vi "KlingerV2 Goto.vi"(0 "VISA Rsrc":refnum<visa-resource-name>="SR530", 1 "Ctrl Refs":T1, 5 "Relatif":bool caption="Relatif/Absolu\n(Absolu)", 7 "UnitDem":u8(ring)=2 caption="Unités" items=["Pas", "mm", "ps"], 9 "PosDem":dbl=1.0 caption="Position dem (pas)" min=-7999999.9 max=7999999.9 step=0.1 format="%#_8f", 11 "error in":errorcluster, 12 "Axe":u8(ring) items=["W", "X", "Y", "Z"]) -> (3 "Erreur":bool, 4 "Pos Init":dbl caption="Position Initiale", 6 "PosErreur":dbl caption="Erreur de\nPositionnement", 8 "Limits":cluster{"PLimit":bool, "NLimit":bool}, 10 "Position Out":dbl format="%#.3f", 14 "Indcomm":string caption="Indicateur de commande", 15 "error out":errorcluster)   [LabVIEW 2019]
doc: "Ce VI envoie une commande de déplacement au controlleur Klinger MC4. \n\nAxe : Sélectionner l'axe sur lequel effectuer le déplacement\n\nAllez à :En mode de déplacement absolu, entrer la position de destination en pas. En mode de déplacement relatif, entrer le nombre de pas à effectuer. Le signe indique la direcetion de déplacement. Valeur accepter :-7 999 999,9 à 7 999 999,9\n\nRelatif/Absolu : Choisi le type de déplacementà effectuer. En mode absolu, le déplacement est effectué par rapport à une position de référence prédéfini. En mode relatif, le déplacement est effectué par rapport à la position actuelle.\n\nLimite + : Indique l'atteinte de l'interrupeur de fin de course positif\n\nLimite - : Indique l'atteinte de l'interrupeur de fin de course négatif\n\nPosition: Indique la position finale"
uses:
  <userlib>/KlingerV2/KlingerV2 Params.ctl
  <userlib>/KlingerV2/KlingerV2 GotoStates.ctl
  <vilib>/Utility/error.llb/DialogType.ctl
panel:
  out "Stopped":bool
  out "NbEssais":i32
  out "Message D'erreur":string
  out "Moving":bool caption="Déplacement\nen cours"
  # "Relatif"
  # "Absolu"
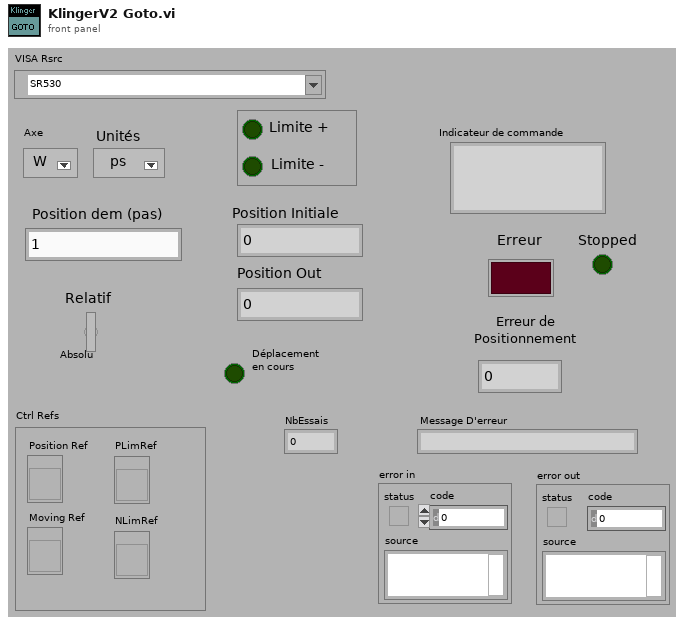
[diagram p1: front panel]
types:
  T1 = cluster{"Position Ref":refnum<vi>, "Moving Ref":refnum<vi>, "PLimRef":refnum<vi>, "NLimRef":refnum<vi>}
  T2 = typedef "KlingerV2 GotoStates.ctl" = enum16{"Dem Pos Init", "Lire Pos Init", "Envoie Comm", "Dem Statut", "Lire Statut", "Attend RQS", "Erreur GPIB", "Dépl incomp", "StopMove", "Dépl comp"}
  T3 = typedef "KlingerV2 Params.ctl" = enum16{"Type", "Origine", "Encodeur", "TypeMouv", "FactConv", "Nom", "CorrParams", "KlingCtrlPar", "Speed", "Acc", "Avance", "Tous"}
  T4 = cluster{"CorrActive":bool, "ErreurLim":dbl, "NbrEssais":i32}
  T5 = typedef "DialogType.ctl" = u16
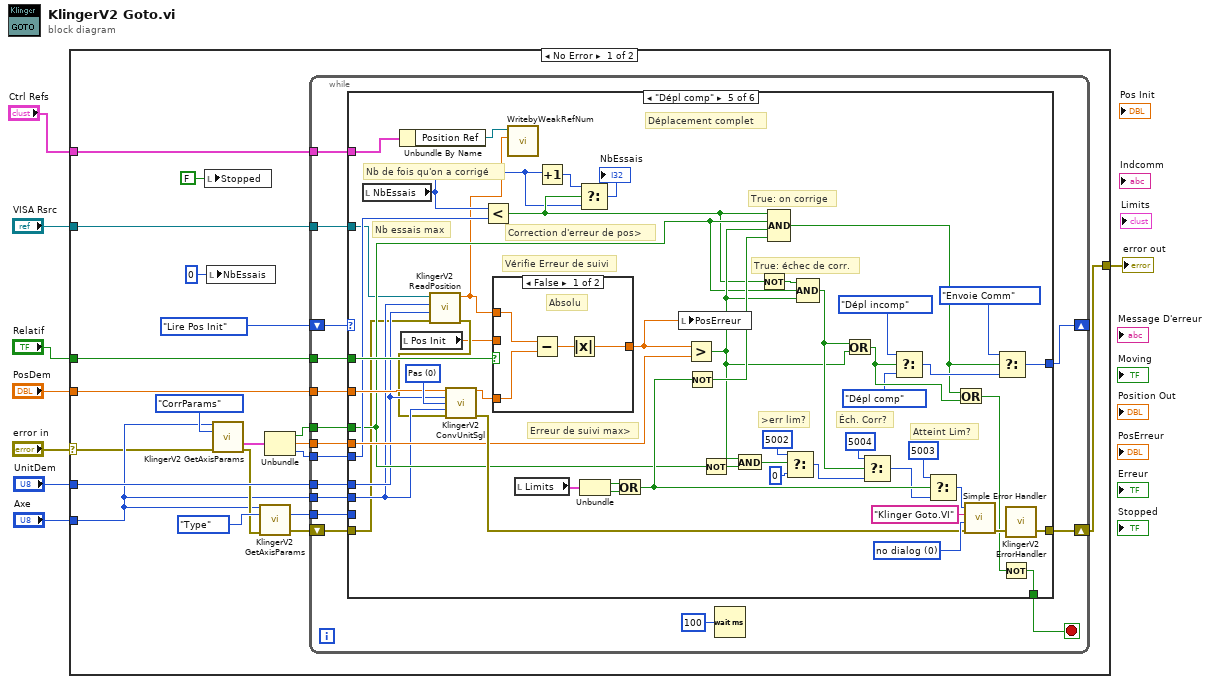
[diagram p0: block diagram]
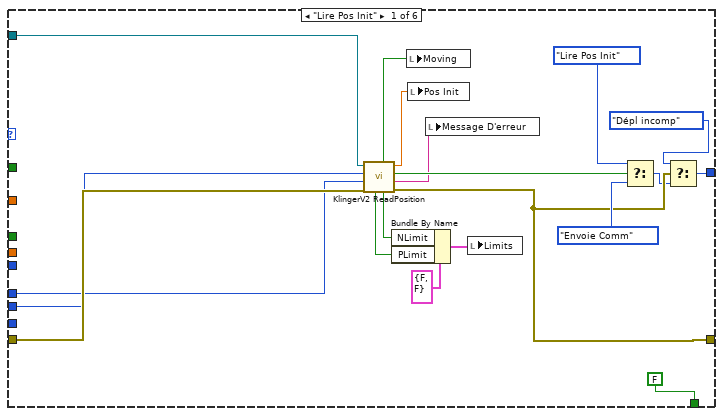
[diagram p2: hidden frame]
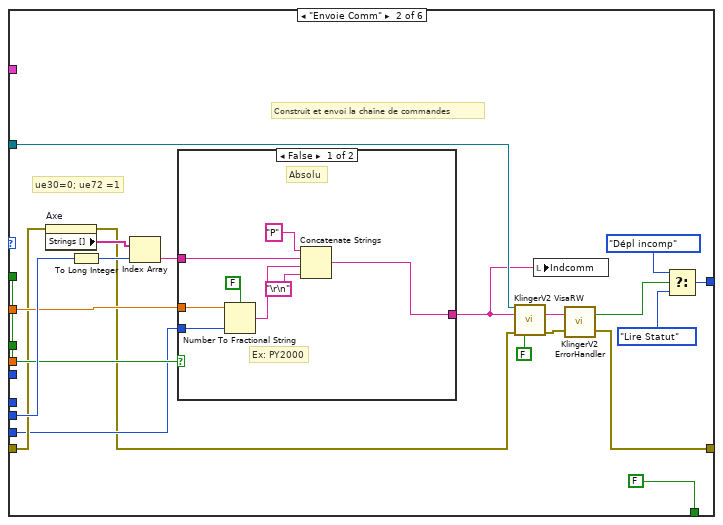
[diagram p3: hidden frame]
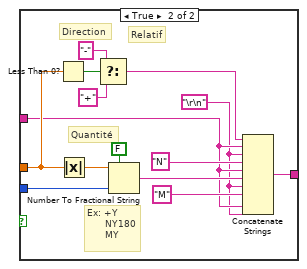
[diagram p4: hidden frame]
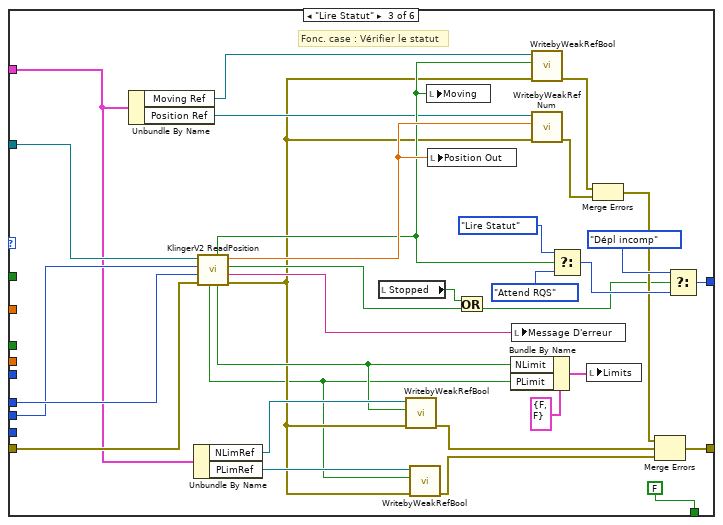
[diagram p5: hidden frame]
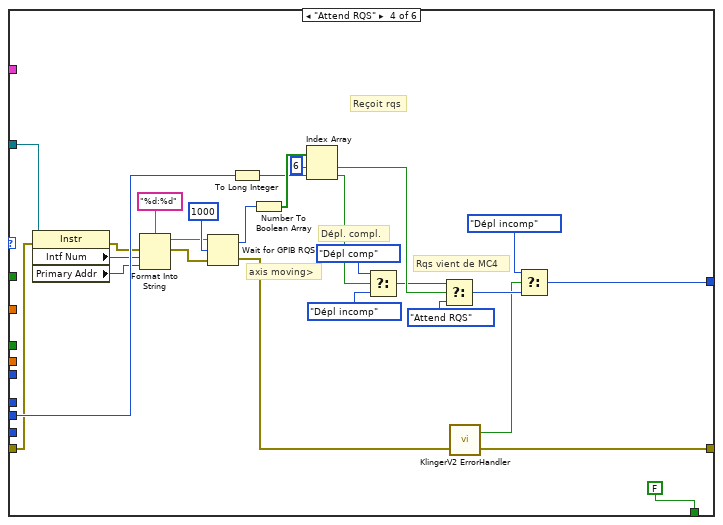
[diagram p6: hidden frame]
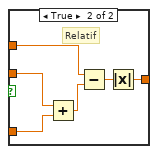
[diagram p7: hidden frame]
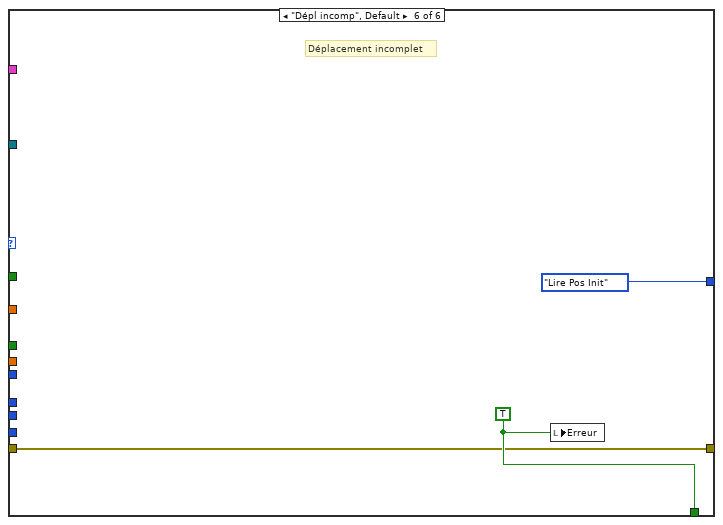
[diagram p8: hidden frame]
diagram:
  n1 = case shown="No Error" "error in" {
    selector: "error in" -> [w10 w230]
    tunnel: [w28 w230] -> w8
    tunnel: "UnitDem" -> [w21 _]
    tunnel: "PosDem" -> [w20 _]
    tunnel: "Relatif" -> [w19 _]
    tunnel: "Axe" -> [w11 _]
    tunnel: "VISA Rsrc" -> [w9 _]
    tunnel: "Ctrl Refs" -> [w14 _]
    frame No Error {
      n2 = local write "Stopped"(FALSE ("Stopped")) -> ()
      n3 = local write "NbEssais"(0 ("Numeric")) -> ()
      n4 = call <userlib>:"KlingerV2 GetAxisParams.vi"("Axe"=w11, "Param"=KlingerV2_Params."CorrParams", "error in"=w10) -> ("CorrParams"=w18:T4, "error out"=w17:errorcluster)  [unwired: 3 in, 8 out]
      n5 = call <userlib>:"KlingerV2 GetAxisParams.vi"("Axe"=w11, "Param"=KlingerV2_Params."Type", "error in"=w17) -> ("Type"=w22:i32, "error out"=w16:errorcluster)  [unwired: 3 in, 8 out]
      n6 = Unbundle(w18) -> ("CorrActive"=w25:bool, "ErreurLim"=w26:dbl, "NbrEssais"=w24:i32)
      n7 = while {
        shift-right: [w43] -> w28
        shift-left: w16 -> [w42]
        tunnel: w11 -> [w41]
        tunnel: w20 -> [w40]
        tunnel: w19 -> [w39]
        shift-right: [w36] -> _
        shift-left: KlingerV2_GotoStates."Lire Pos Init" ("KlingerV2 GotoStates") -> [w37]
        tunnel: w24 -> [w35]
        tunnel: w21 -> [w34]
        tunnel: w26 -> [w33]
        tunnel: w25 -> [w32]
        tunnel: w22 -> [w31]
        tunnel: w9 -> [w30]
        tunnel: w14 -> [w29]
        stop <- w44 stop-if-true
        n8 = case shown="\"Dépl comp\"" w37 {
          tunnel: [FALSE FALSE FALSE FALSE w212 w229] -> w44
          tunnel: [w47 w76 w112 w138 w211 w228] -> w43
          tunnel: w42 -> [w60 w73 w133 w146 w168 w228]
          tunnel: w41 -> [w56 w80 w130 w164 w169 _]
          tunnel: w40 -> [_ w74 _ _ w203 _]
          tunnel: w39 -> [_ w78 _ _ w216 _]
          tunnel: [w48 w77 w136 w139 w204 KlingerV2_GotoStates."Lire Pos Init" ("KlingerV2 GotoStates")] -> w36
          tunnel: w35 -> [_ _ _ _ w179 _]
          tunnel: w34 -> [w57 _ w131 _ w170 _]
          tunnel: w33 -> [_ _ _ _ w189 _]
          tunnel: w32 -> [_ _ _ _ w178 _]
          tunnel: w31 -> [_ w72 _ _ _ _]
          tunnel: w30 -> [w58 w71 w127 w148 w173 _]
          tunnel: w29 -> [_ _ w120 _ w172 _]
          frame "Lire Pos Init" {
            n9 = call <userlib>:"KlingerV2 ReadPosition.vi"("error in"=w60, "UnitDem"=w57, "Axe"=w56, "VISA Rsrc"=w58) -> ("error out"=w47:errorcluster, "Cont Error"=w61:string, "Statut"=w62:bool, "Position"=w59:dbl, "NLimit"=w52:bool, "Moving"=w55:bool, "PLimit"=w53:bool)  [unwired: 1 in]
            n10 = Bundle By Name(cluster=cluster{"PLimit":bool, "NLimit":bool} {"PLimit"=FALSE, "NLimit"=FALSE} ("Limits"), "NLimit"=w52, "PLimit"=w53) -> (w51:cluster{"PLimit":bool, "NLimit":bool})
            n11 = local write "Moving"(w55) -> ()
            n12 = local write "Pos Init"(w59) -> ()
            n13 = local write "Message D'erreur"(w61) -> ()
            n14 = local write "Limits"(w51) -> ()
            n15 = Select(t=KlingerV2_GotoStates."Lire Pos Init" ("KlingerV2 GotoStates"), s=w62, f=KlingerV2_GotoStates."Envoie Comm" ("KlingerV2 GotoStates")) -> (s? t:f=w46:T2)
            n16 = Select(t=KlingerV2_GotoStates."Dépl incomp" ("KlingerV2 GotoStates"), s=w47, f=w46) -> (s? t:f=w48:T2)
          }
          frame "Envoie Comm" {
            # "ue30=0; ue72 =1"
            # "Construit et envoi la chaîne de commandes"
            n17 = property on="Axe" class="Ring (strict)"(error in=w73) -> (error out=w70:errorcluster, "Strings []"=w83:string[])  [unwired: 1 in, 1 out]
            n18 = To Long Integer(number=w80) -> (32bit integer=w79:i32)
            n19 = Index Array(array=w83, index=w79) -> (element=w82:string)
            n20 = case shown="False" w78 {
              tunnel: w74 -> [w91 w103]
              tunnel: w82 -> [w88 w95]
              tunnel: [w86 w93] -> w69
              tunnel: w72 -> [w84 w92]
              frame False {
                # "Ex: PY2000"
                # "Absolu"
                n21 = Number To Fractional String(use system decimal point (T)=FALSE, number=w91, precision (6)=w84) -> (F-format string=w90:string)  [unwired: 1 in]
                n22 = Concatenate Strings("P", w88, w90, "\r\n") -> (w86:string)
              }
              frame True {
                w94 = "\r\n"
                # "Quantité"
                # "Direction"
                # "Ex: +Y\n      NY180\n      MY"
                # "Relatif"
                n23 = Less Than 0?(x=w103) -> (x < 0?=w102:bool)
                n24 = Absolute Value(x=w103) -> (abs(x)=w105:dbl)
                n25 = Select(t="-", s=w102, f="+") -> (s? t:f=w99:string)
                n26 = Number To Fractional String(use system decimal point (T)=FALSE, number=w105, precision (6)=w92) -> (F-format string=w97:string)  [unwired: 1 in]
                n27 = Concatenate Strings(w99, w95, w94, "N", w95, w97, w94, "M", w95, w94) -> (w93:string)
              }
            }
            n28 = call <userlib>:"KlingerV2 VisaRW.vi"("VISA Rsrc"=w71, "ChaineCom"=w69, "error in (no error)"=w70, "Lecture?(T)"=FALSE) -> ("ChaineRep"=w67:string, "error out"=w68:errorcluster)  [unwired: 7 in, 3 out]
            n29 = local write "Indcomm"(w69) -> ()
            n30 = call <userlib>:"KlingerV2 ErrorHandler.vi"("error in (no error)"=w68, "Message D'erreur"=w67) -> ("error out"=w76:errorcluster, "Erreur"=w75:bool)
            n31 = Select(t=KlingerV2_GotoStates."Dépl incomp" ("KlingerV2 GotoStates"), s=w75, f=KlingerV2_GotoStates."Lire Statut" ("KlingerV2 GotoStates")) -> (s? t:f=w77:T2)
          }
          frame "Lire Statut" {
            # "Fonc. case : Vérifier le statut"
            n32 = Unbundle By Name(w120) -> ("Moving Ref"=w124:refnum<vi>, "Position Ref"=w123:refnum<vi>)
            n33 = Unbundle By Name(w120) -> ("NLimRef"=w119:refnum<vi>, "PLimRef"=w118:refnum<vi>)
            n34 = call <userlib>:"KlingerV2 ReadPosition.vi"("error in"=w133, "UnitDem"=w131, "Axe"=w130, "VISA Rsrc"=w127) -> ("error out"=w116:errorcluster, "Cont Error"=w132:string, "Statut"=w134:bool, "Position"=w129:dbl, "NLimit"=w117:bool, "Moving"=w128:bool, "PLimit"=w115:bool)  [unwired: 1 in]
            n35 = local read "Stopped"() -> (w107:bool)
            n36 = call <userlib>:"WritebyWeakRefBool.vi"("error in"=w116, "Valeur"=w117, "Control Ref"=w119) -> ("error out"=w110:errorcluster)  [unwired: 8 in]
            n37 = call <userlib>:"WritebyWeakRefBool.vi"("error in"=w116, "Valeur"=w115, "Control Ref"=w118) -> ("error out"=w109:errorcluster)  [unwired: 8 in]
            n38 = local write "Moving"(w128) -> ()
            n39 = local write "Position Out"(w129) -> ()
            n40 = Or(x=w107, y=w134) -> (x .or. y?=w108:bool)
            n41 = Bundle By Name(cluster=cluster{"PLimit":bool, "NLimit":bool} {"PLimit"=FALSE, "NLimit"=FALSE} ("Limits"), "NLimit"=w117, "PLimit"=w115) -> (w125:cluster{"PLimit":bool, "NLimit":bool})
            n42 = local write "Message D'erreur"(w132) -> ()
            n43 = call <userlib>:"WritebyWeakRefBool.vi"("error in"=w116, "Valeur"=w128, "Control Ref"=w124) -> ("error out"=w113:errorcluster)  [unwired: 8 in]
            n44 = call <userlib>:"WritebyWeakRefNum.vi"("error in"=w116, "Valeur"=w129, "Control Ref"=w123) -> ("error out"=w114:errorcluster)  [unwired: 8 in]
            n45 = Select(t=KlingerV2_GotoStates."Lire Statut" ("KlingerV2 GotoStates"), s=w128, f=KlingerV2_GotoStates."Attend RQS" ("KlingerV2 GotoStates")) -> (s? t:f=w135:T2)
            n46 = local write "Limits"(w125) -> ()
            n47 = Merge Errors(w113, w114) -> (w111:errorcluster)
            n48 = Merge Errors(w111, w110, w109) -> (w112:errorcluster)
            n49 = Select(t=KlingerV2_GotoStates."Dépl incomp" ("KlingerV2 GotoStates"), s=w108, f=w135) -> (s? t:f=w136:T2)
          }
          frame "Attend RQS" {
            # "axis moving>"
            # "Dépl. compl."
            # "Rqs vient de MC4"
            # "Reçoit rqs"
            n50 = property class="Instr"(reference=w148, error in=w146) -> (error out=w143:errorcluster, "Intf Num"=w145:u16, "Primary Addr"=w144:u16)  [unwired: 1 out]
            n51 = Format Into String(format string="%d:%d" ("chaîne de format"), error in=w143, w145, w144) -> (resulting string=w142:string, error out=w141:errorcluster)  [unwired: 1 in]
            n52 = Wait for GPIB RQS(2:w141, 3:1000 ("timeout (25000 ms)"), 4:w142) -> (0:w150:errorcluster, 1:w149:i16)
            n53 = To Long Integer(number=w164) -> (32bit integer=w159:i32)
            n54 = Number To Boolean Array(number=w149) -> (Boolean array=w163:bool[])
            n55 = Index Array(array=w163, index #1=6 ("index"), index #2=w159) -> (element #1=w161:bool, element #2=w158:bool)
            n56 = Select(t=KlingerV2_GotoStates."Dépl comp" ("KlingerV2 GotoStates"), s=w158, f=KlingerV2_GotoStates."Dépl incomp" ("KlingerV2 GotoStates")) -> (s? t:f=w157:T2)
            n57 = Select(t=w157, s=w161, f=KlingerV2_GotoStates."Attend RQS" ("KlingerV2 GotoStates")) -> (s? t:f=w156:T2)
            n58 = call <userlib>:"KlingerV2 ErrorHandler.vi"("error in (no error)"=w150) -> ("error out"=w138:errorcluster, "Erreur"=w155:bool)  [unwired: 1 in]
            n59 = Select(t=KlingerV2_GotoStates."Dépl incomp" ("KlingerV2 GotoStates"), s=w155, f=w156) -> (s? t:f=w139:T2)
          }
          frame "Dépl comp" {
            w210 = u8 0 items=["Pas", "mm", "ps"] ("UnitAct")
            w214 = T5 0 items=["no dialog", "OK message", "continue or stop message", "OK message + warnings", "continue/stop + warnings"] ("type of dialog (OK msg:1)")
            # "Nb essais max"
            # "Correction d'erreur de pos>"
            # "Erreur de suivi max>"
            # ">err lim?"
            # "Éch. Corr?"
            # "Atteint Lim?"
            # "Nb de fois qu'on a corrigé"
            # "True: échec de corr."
            # "True: on corrige"
            # "Vérifie Erreur de suivi"
            # "Déplacement complet"
            n60 = local read "NbEssais"() -> (w176:i32)
            n61 = Unbundle By Name(w172) -> ("Position Ref"=w171:refnum<vi>)
            n62 = local read "Pos Init"() -> (w166:dbl)
            n63 = call <userlib>:"KlingerV2 ReadPosition.vi"("error in"=w168, "UnitDem"=w170, "Axe"=w169, "VISA Rsrc"=w173) -> ("error out"=w167:errorcluster, "Position"=w165:dbl)  [unwired: 1 in, 5 out]
            n64 = call <userlib>:"KlingerV2 ConvUnitSgl.vi"("ParamAct"=w203, "UnitDem"=w170, "UnitAct"=w210, "Axe"=w169, "error in"=w167) -> ("ParamDem"=w209:dbl, "error out"=w190:errorcluster)  [unwired: 9 in]
            n65 = Less?(x=w176, y=w179) -> (x < y?=w177:bool)
            n66 = case shown="False" w216 {
              tunnel: w166 -> [_ w225]
              tunnel: w209 -> [w220 w224]
              tunnel: [w219 w222] -> w208
              tunnel: w165 -> [w218 w221]
              frame False {
                # "Absolu"
                n67 = Subtract(x=w218, y=w220) -> (x-y=w217:dbl)
                n68 = Absolute Value(x=w217) -> (abs(x)=w219:dbl)
              }
              frame True {
                # "Relatif"
                n69 = Add(x=w225, y=w224) -> (x+y=w226:dbl)
                n70 = Subtract(x=w221, y=w226) -> (x-y=w223:dbl)
                n71 = Absolute Value(x=w223) -> (abs(x)=w222:dbl)
              }
            }
            n72 = call <userlib>:"WritebyWeakRefNum.vi"("Valeur"=w165, "Control Ref"=w171) -> ()  [unwired: 9 in, 1 out]
            n73 = local read "Limits"() -> (w188:cluster{"PLimit":bool, "NLimit":bool})
            n74 = Increment(x=w176) -> (x+1=w175:i32)
            n75 = Select(t=w175, s=w177, f=w176) -> (s? t:f=→"NbEssais":i32)
            n76 = Unbundle(w188) -> ("PLimit"=w187:bool, "NLimit"=w186:bool)
            n77 = Or(x=w187, y=w186) -> (x .or. y?=w200:bool)
            n78 = local write "PosErreur"(w208) -> ()
            n79 = Greater?(x=w208, y=w189) -> (0:w182:bool)
            n80 = Not(x=w200) -> (.not. x?=w206:bool)
            n81 = Not(x=w178) -> (.not. x?=w181:bool)
            n82 = And(x=w182, y=w181) -> (x .and. y?=w180:bool)
            n83 = Not(x=w177) -> (.not. x?=w202:bool)
            n84 = Compound Arithmetic op=AND(w177, w178, w182, w206) -> (w192:bool)
            n85 = Select(t=5002 ("error code (no error:0)"), s=w180, f=0 ("error code (no error:0)")) -> (s? t:f=w196:i32)
            n86 = Compound Arithmetic op=AND(w202, w178, w182) -> (w197:bool)
            n87 = Or(x=w197, y=w182) -> (x .or. y?=w193:bool)
            n88 = Select(t=5004 ("error code (no error:0)"), s=w197, f=w196) -> (s? t:f=w194:i32)
            n89 = Select(t=KlingerV2_GotoStates."Dépl incomp" ("KlingerV2 GotoStates"), s=w193, f=KlingerV2_GotoStates."Dépl comp" ("KlingerV2 GotoStates")) -> (s? t:f=w205:T2)
            n90 = Select(t=5003, s=w200, f=w194) -> (s? t:f=w198:i32)
            n91 = Or(x=w192, y=w193) -> (x .or. y?=w191:bool)
            n92 = call <vilib>:"Simple Error Handler.vi"("error code (no error:0)"=w198, "error source (\" \")"="Klinger Goto.VI" ("error source (\" \")"), "type of dialog (OK msg:1)"=w214, "error in (no error)"=w190) -> ("error out"=w215:errorcluster)  [unwired: 1 in, 4 out]
            n93 = Select(t=KlingerV2_GotoStates."Envoie Comm" ("KlingerV2 GotoStates"), s=w192, f=w205) -> (s? t:f=w204:T2)
            n94 = Not(x=w191) -> (.not. x?=w212:bool)
            n95 = call <userlib>:"KlingerV2 ErrorHandler.vi"("error in (no error)"=w215) -> ("error out"=w211:errorcluster)  [unwired: 1 in, 1 out]
          }
          frame "Dépl incomp", Default {
            w229 = TRUE
            # "Déplacement incomplet"
            n96 = local write "Erreur"(w229) -> ()
          }
        }
        n97 = Wait (ms)(milliseconds to wait=u32 100) -> ()  [unwired: 1 out]
      }
    }
    frame Error {
    }
  }
  "error out" <- w8
